vi "Edge Detect.vi"() -> ()   [LabVIEW 2019]
uses:
  <userlib>/Onshape/_SubVI/Cluster.ctl
  <userlib>/IoT Devices/_subVIs/HTTPComm.ctl
  <userlib>/Onshape/_SubVI/z did wid and eid.vi
  <userlib>/OnshapeFeatureFunctions/Onshape Feature Funcrions/_SubVI/FS Sketch Polyline.vi
panel:
  in  "Scaling Factor":dbl
  out "Comm":T1
  out "Device Out":T2
  in  "Image Path":path=path "/Users/milandahal/Desktop/a.png"
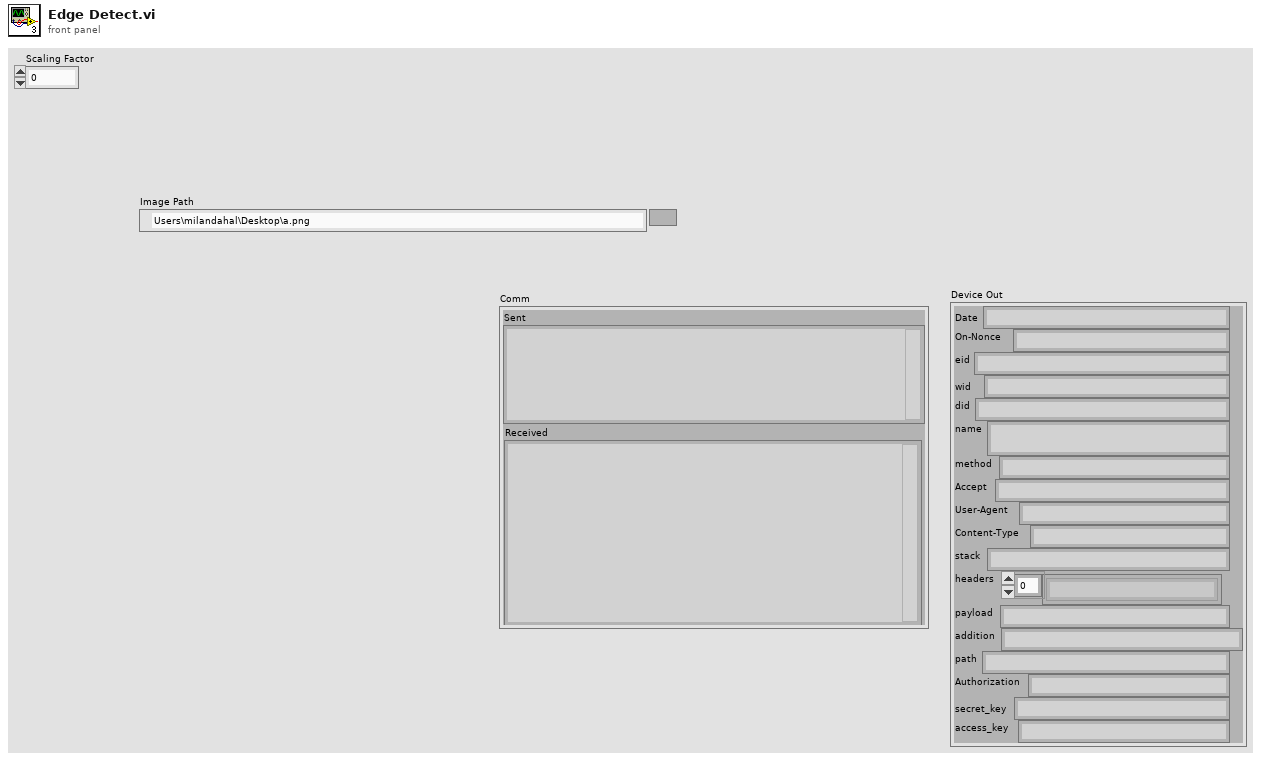
[diagram p1: front panel]
types:
  T1 = typedef "HTTPComm.ctl" = cluster{"url":string, "sent headers":string, "sent body":string, "headers":string, "body":string, "Sent":string, "Received":string}
  T2 = typedef "Cluster.ctl" = cluster{"Date":string, "On-Nonce":string, "eid":string, "wid":string, "did":string, "name":string, "method":string, "Accept":string, "User-Agent":string, "Content-Type":string, "stack":string, "headers":string[], "payload":string, "addition":string, "path":string, "Authorization":string, "secret_key":string, "access_key":string}
  T3 = typedef "QT_Image.ctl" = cluster{"Width":i32, "Height":i32, "Depth":i32, "data":u8[], "Compressed data":u8[], "Color table":u32[], "Duration":i32, "Options":i32, "Timestamp":i32, "ID":i32, "Reserved":i32, "Dialogs":u32}
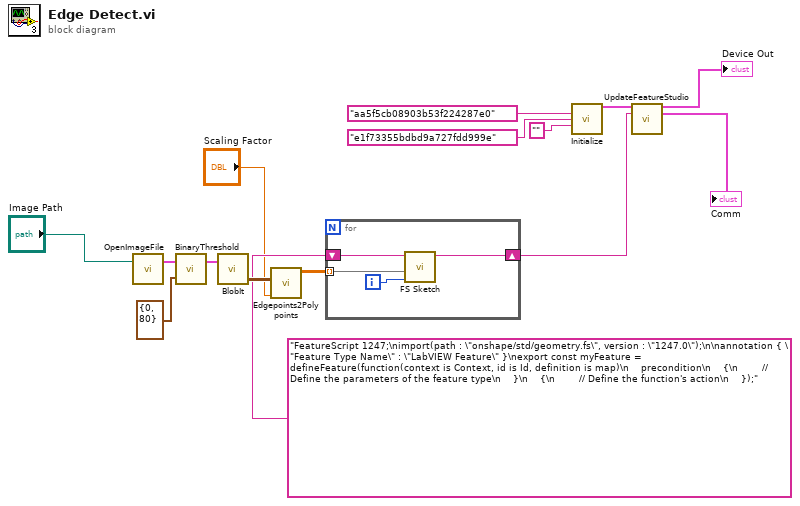
[diagram p0: block diagram]
diagram:
  n1 = call <userlib>:"OpenImageFile.vi"("selected path"="Image Path") -> ("Image Out"=w6:T3)  [unwired: 2 in]
  n2 = call <userlib>:"BinaryThreshold.vi"("threshold"=cluster{u8, u8} {0, 80}, "Image In"=w6) -> ("Image Out"=w5:T3)  [unwired: 1 in]
  n3 = call <userlib>:"BlobIt.vi"("Image in"=w5) -> ("Array 2"=w15:cluster{"Row":i32, "Col":i32}[][])  [unwired: 1 in, 2 out]
  n4 = call <userlib>:"Edgepoints2Polypoints.vi"("Scaling Factor"="Scaling Factor", "Edgepoints In"=w15) -> ("Polyline Out"=w14:dbl[][][])  [unwired: 9 in]
  n5 = for {
    tunnel: w14 -> [w19] mode=indexing
    shift-right: [w16] -> w9
    shift-left: "FeatureScript 1247;\nimport(path : \"onshape/std/geometry.fs\", version : \"1247.0\");\n\nannotation { \"Feature Type Name\" : \"LabVIEW Feature\" }\nexport const myFeature = defineFeature(function(context is Context, id is Id, definition is map)\n    precondition\n    {\n        // Define the parameters of the feature type\n    }\n    {\n        // Define the function's action\n    });" ("Feature In") -> [w17]
    i -> [w18]
    n6 = call-poly <userlib>:"FS Sketch.vi"("Sketch #"=w18, "Polyline Points"=w19, "Feature In"=w17) -> ("Feature Out"=w16:string)  [unwired: 8 in]
  }
  n7 = call-poly <userlib>:"Initialize.vi"("did"="aa5f5cb08903b53f224287e0", "wid"="e1f73355bdbd9a727fdd999e", "eid"="") -> ("Device Out"=w10:T2)  [unwired: 11 in, 1 out]
  n8 = call <userlib>:"UpdateFeatureStudio.vi"("Device In"=w10, "FeatureScript"=w9) -> ("Device Out"=→"Device Out":T2, "Comm"=→"Comm":T1)  [unwired: 11 in, 1 out]
